vi "Integrate_diag_optional.vi"(6 "Continous Lock-in":bool, 7 "Cutoff Frequency":dbl, 8 "Ref Sine":dbl[](array[numeric]), 9 "Processed LD values":dbl[](array[numeric]), 10 "Ref Cosine":dbl[](array[numeric]), 11 "Window (s)":dbl) -> (0 "dTheta":dbl format="%0.2f", 1 "Theta":dbl format="%0.2f", 2 "dR":dbl format="%0.5f", 3 "Lockin R":dbl format="%0.5f", 4 "Phase (deg)":waveform(dbl)(graph), 5 "LockIN R (cont/disc)":waveform(dbl)(graph))   [LabVIEW 2013]
uses:
  <vilib>/Analysis/8numeric.llb/1D Numeric Integration.vi
  <vilib>/express/express arith-compare/Formula/XNode/ExpressFormulaBlockNode.xnode
  <vilib>/Analysis/NI_AALPro.lvlib
  <vilib>/Analysis/NI_AALBase.lvlib
panel:
  in  "Processed LD time values":dbl[](array[numeric])
  out "X":dbl[](graph)
  out "Y":dbl[](graph)
  out "theta":dbl[](array[numeric])
  out "r":dbl[](array[numeric])
  out "LockIn Theta Array":dbl[](array[numeric])
  out "Lock in X,Y,R (Vrms) time":cluster{dbl[], "Result":dbl[]}[](array[cluster])
  out "Lockin Theta":cluster{dbl[], "Result":dbl[]}
  out "LockIn R (Vrms)":cluster{dbl[], "Result":dbl[]}
  out "LockIn R (Vrms) array":dbl[](array[numeric])
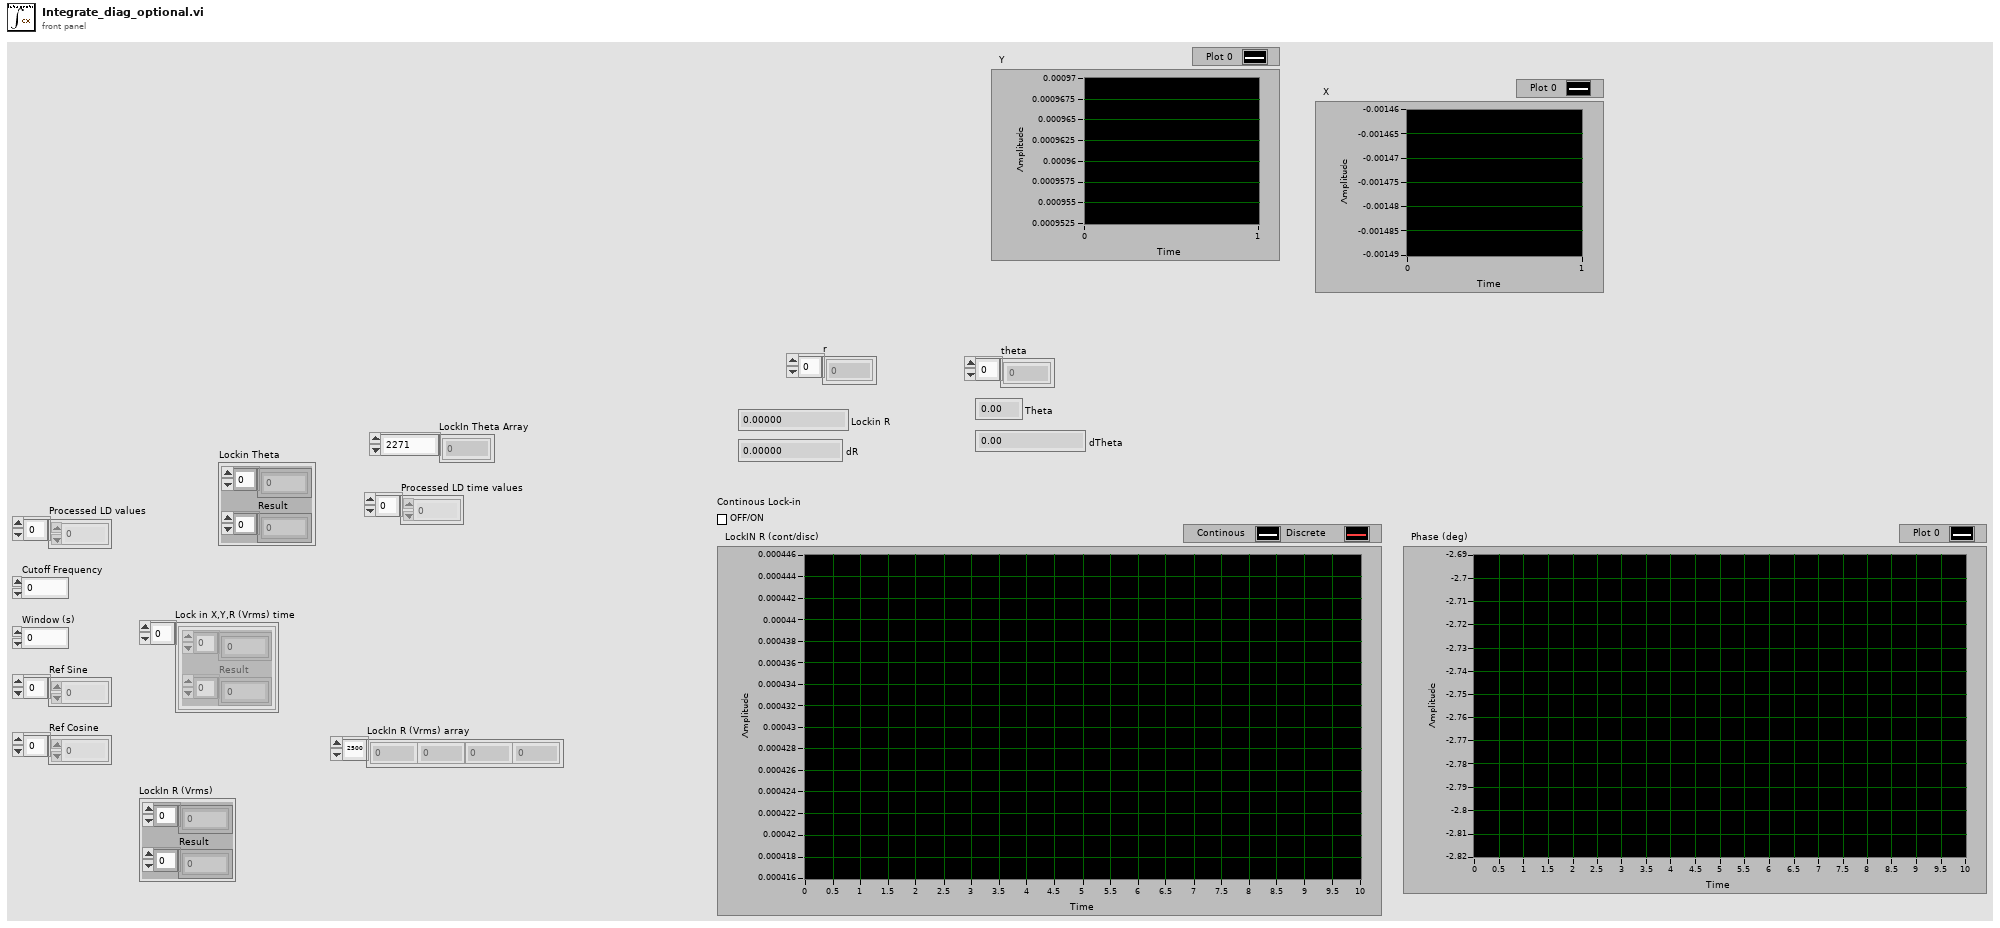
[diagram p1: front panel]
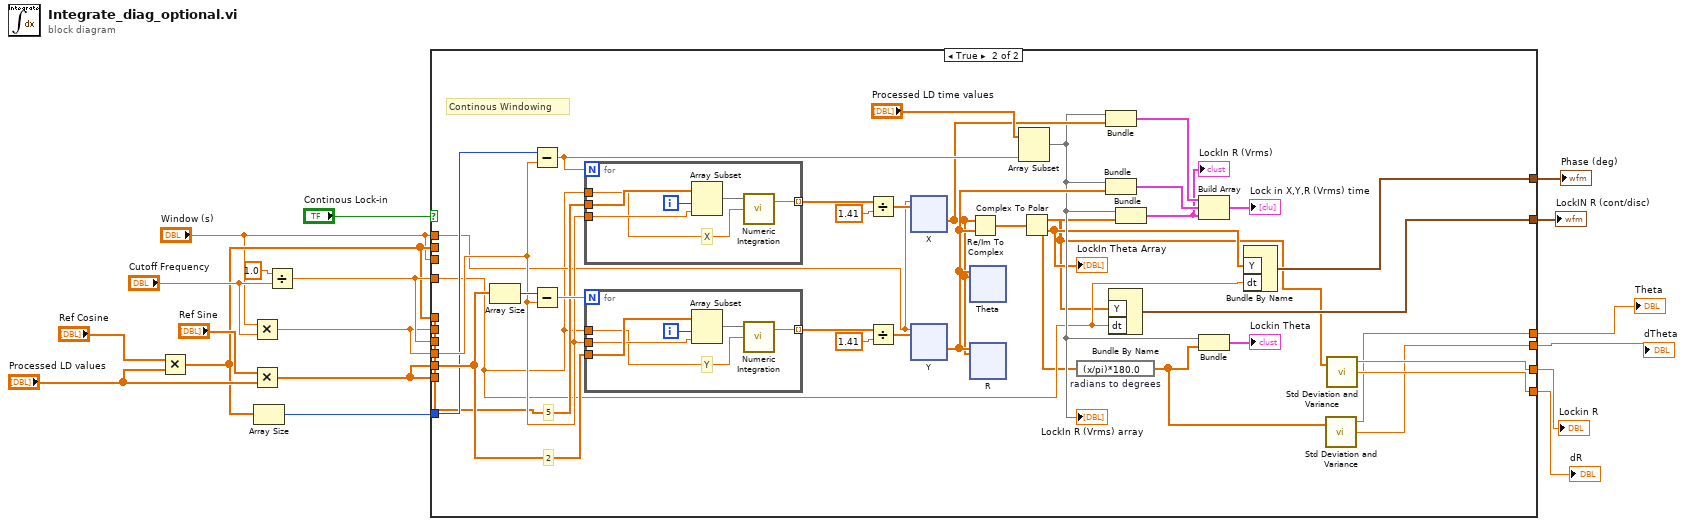
[diagram p0: block diagram]
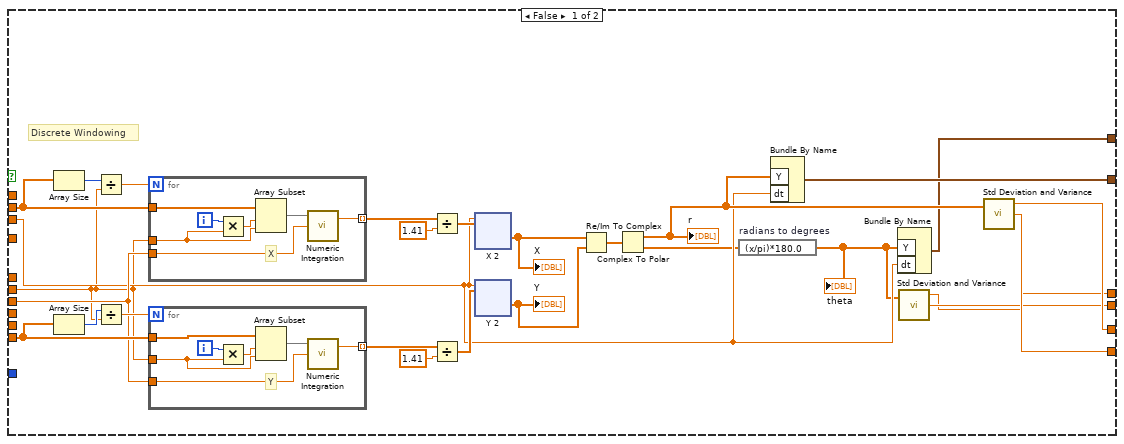
[diagram p2: hidden frame]
diagram:
  n1 = Multiply(x="Ref Cosine", y="Processed LD values") -> (x*y=w8:dbl[])
  n2 = Multiply(x="Window (s)", y="Cutoff Frequency") -> (x*y=w10:dbl)
  n3 = Multiply(x="Ref Sine", y="Processed LD values") -> (x*y=w11:dbl[])
  n4 = Array Size(array=w8) -> (size(s)=w9:i32)
  n5 = Divide(x=1.0, y="Cutoff Frequency") -> (x/y=w12:dbl)
  n6 = case shown="True" "Continous Lock-in" {
    tunnel: w11 -> [w45 _]
    tunnel: w8 -> [w44 _]
    tunnel: w12 -> [w31 _]
    tunnel: "Window (s)" -> [w30 _]
    tunnel: w10 -> [w29 _]
    tunnel: [w24 w99] -> w13
    tunnel: w12 -> [_ w90]
    tunnel: w11 -> [_ w104]
    tunnel: w10 -> [_ w103]
    tunnel: w9 -> [_ w102]
    tunnel: w8 -> [_ w101]
    tunnel: "Window (s)" -> [_ w100]
    tunnel: [w23 w93] -> w6
    tunnel: [w22 w94] -> w5
    tunnel: [w21 w91] -> w4
    tunnel: [w20 w92] -> w2
    tunnel: [w19 w89] -> w1
    frame False {
      # "Discrete Windowing"
      n7 = Array Size(array=w44) -> (size(s)=w42:i32)
      n8 = Array Size(array=w45) -> (size(s)=w43:i32)
      n9 = Divide(x=w42, y=w29) -> (x/y=w40:dbl)
      n10 = Divide(x=w43, y=w29) -> (x/y=w41:dbl)
      n11 = for {
        N: w40 -> [_]
        tunnel: w44 -> [w78]
        tunnel: w29 -> [w72]
        tunnel: [w76] -> w36 mode=indexing
        tunnel: w31 -> [w75]
        i -> [w74]
        # "X"
        n12 = Multiply(x=w74, y=w72) -> (x*y=w73:dbl)
        n13 = Array Subset(array=w78, index=w73, length=w72) -> (w77:dbl[])
        n14 = call-poly <vilib>:"Numeric Integration.vi"("dt"=w75, "Input Array"=w77) -> ("result"=w76:dbl)  [unwired: 1 in, 1 out]
      }
      n15 = for {
        N: w41 -> [_]
        tunnel: w45 -> [w85]
        tunnel: w29 -> [w79]
        tunnel: [w83] -> w39 mode=indexing
        tunnel: w31 -> [w80]
        i -> [w81]
        # "Y"
        n16 = Multiply(x=w81, y=w79) -> (x*y=w82:dbl)
        n17 = Array Subset(array=w85, index=w82, length=w79) -> (w84:dbl[])
        n18 = call-poly <vilib>:"Numeric Integration.vi"("dt"=w80, "Input Array"=w84) -> ("result"=w83:dbl)  [unwired: 1 in, 1 out]
      }
      n19 = Divide(x=w36, y=1.41) -> (x/y=w33:dbl[])
      n20 = Divide(x=w39, y=1.41) -> (x/y=w34:dbl[])
      n21 = xnode "X 2"("X1"=w30, "X2"=w33) -> ("Result"=w25:dbl[])  [unwired: 1 in, 1 out]
      "X" <- w25
      n22 = xnode "Y 2"("X1"=w30, "X2"=w34) -> ("Result"=w26:dbl[])  [unwired: 1 in, 1 out]
      "Y" <- w26
      n23 = Re/Im To Complex(1:w26, 2:w25) -> (0:w35:cdb[])
      n24 = Complex To Polar(r * e^(i*theta)=w35) -> (r=w32:dbl[], theta=w28:dbl[])
      "r" <- w32
      n25 = expression code="(x/pi)*180.0" "radians to degrees"(w28) -> (w27:dbl[])
      "theta" <- w27
      n26 = Bundle By Name("Y"=w32, "dt"=w30) -> (w24:waveform(dbl))  [unwired: 1 in]
      n27 = Bundle By Name("Y"=w27, "dt"=w30) -> (w19:waveform(dbl))  [unwired: 1 in]
      n28 = call <vilib>:"Std Deviation and Variance.vi"("X"=w27) -> ("mean"=w20:dbl, "standard deviation"=w21:dbl)  [unwired: 1 in, 1 out]
      n29 = call <vilib>:"Std Deviation and Variance.vi"("X"=w32) -> ("mean"=w22:dbl, "standard deviation"=w23:dbl)  [unwired: 1 in, 1 out]
    }
    frame True {
      # "5"
      # "2"
      # "Continous Windowing"
      n30 = Array Size(array=w104) -> (size(s)=w105:i32)
      n31 = Subtract(x=w102, y=w103) -> (x-y=w115:dbl)
      n32 = Subtract(x=w105, y=w103) -> (x-y=w116:dbl)
      n33 = for {
        N: w115 -> [_]
        tunnel: w101 -> [w181]
        tunnel: w103 -> [w183]
        tunnel: [w179] -> w113 mode=indexing
        tunnel: w90 -> [w178]
        i -> [w182]
        # "X"
        n34 = Array Subset(array=w181, index=w182, length=w183) -> (w180:dbl[])
        n35 = call-poly <vilib>:"Numeric Integration.vi"("dt"=w178, "Input Array"=w180) -> ("result"=w179:dbl)  [unwired: 1 in, 1 out]
      }
      n36 = for {
        N: w116 -> [_]
        tunnel: w104 -> [w177]
        tunnel: w103 -> [w176]
        tunnel: [w173] -> w110 mode=indexing
        tunnel: w90 -> [w172]
        i -> [w175]
        # "Y"
        n37 = Array Subset(array=w177, index=w175, length=w176) -> (w174:dbl[])
        n38 = call-poly <vilib>:"Numeric Integration.vi"("dt"=w172, "Input Array"=w174) -> ("result"=w173:dbl)  [unwired: 1 in, 1 out]
      }
      n39 = Divide(x=w113, y=1.41) -> (x/y=w112:dbl[])
      n40 = Divide(x=w110, y=1.41) -> (x/y=w109:dbl[])
      n41 = xnode "X"("X1"=w100, "X2"=w112) -> ("Result"=w106:dbl[])  [unwired: 1 in, 1 out]
      n42 = xnode "Y"("X1"=w100, "X2"=w109) -> ("Result"=w107:dbl[])  [unwired: 1 in, 1 out]
      n43 = Re/Im To Complex(1:w107, 2:w106) -> (0:w108:cdb[])
      n44 = xnode "Theta"("X1"=w107, "X2"=w106) -> ()  [unwired: 1 in, 2 out]
      n45 = xnode "R"("X1"=w107, "X2"=w106) -> ()  [unwired: 1 in, 2 out]
      n46 = Array Subset(array="Processed LD time values", length=w115) -> (w95:dbl[])  [unwired: 1 in]
      "LockIn R (Vrms) array" <- w95
      n47 = Complex To Polar(r * e^(i*theta)=w108) -> (r=w87:dbl[], theta=w88:dbl[])
      "LockIn Theta Array" <- w88
      n48 = expression code="(x/pi)*180.0" "radians to degrees"(w88) -> (w86:dbl[])
      n49 = Bundle(w95, "Result"=w106) -> (w117:cluster{dbl[], "Result":dbl[]})  [unwired: 1 in]
      n50 = Bundle(w95, "Result"=w107) -> (w118:cluster{dbl[], "Result":dbl[]})  [unwired: 1 in]
      n51 = Bundle By Name("Y"=w87, "dt"=w90) -> (w99:waveform(dbl))  [unwired: 1 in]
      n52 = Bundle(w95, w87) -> (w96:cluster{dbl[], dbl[]})  [unwired: 1 in]
      "LockIn R (Vrms)" <- w96
      n53 = Build Array(w117, w118, w96) -> (→"Lock in X,Y,R (Vrms) time":cluster{dbl[], "Result":dbl[]}[])
      n54 = Bundle(w95, w86) -> (→"Lockin Theta":cluster{dbl[], dbl[]})  [unwired: 1 in]
      n55 = Bundle By Name("Y"=w88, "dt"=w90) -> (w89:waveform(dbl))  [unwired: 1 in]
      n56 = call <vilib>:"Std Deviation and Variance.vi"("X"=w86) -> ("mean"=w92:dbl, "standard deviation"=w91:dbl)  [unwired: 1 in, 1 out]
      n57 = call <vilib>:"Std Deviation and Variance.vi"("X"=w87) -> ("mean"=w94:dbl, "standard deviation"=w93:dbl)  [unwired: 1 in, 1 out]
    }
  }
  "LockIN R (cont/disc)" <- w13
  "Lockin R" <- w5
  "dR" <- w6
  "dTheta" <- w4
  "Theta" <- w2
  "Phase (deg)" <- w1
